vi "Writeini.vi"(10 "Number Sample for avarage AF":i32, 11 "data":waveform(dbl)[](array[waveform])) -> ()   [LabVIEW 2017]
uses:
  <vilib>/measure/matone.llb/Harmonic Distortion Analyzer N Chan.vi
  <vilib>/measure/matone.llb/Extract Single Tone Information N Chan.vi
  <vilib>/Utility/config.llb/Write Key (Double).vi
  <vilib>/Utility/config.llb/Write Key (Boolean).vi
  <vilib>/Utility/config.llb/NI_LVConfig.lvlib
  <vilib>/measure/NI_MAPro.lvlib
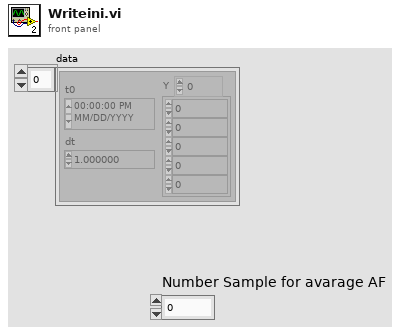
[diagram p1: front panel]
types:
  T1 = typedef "NI_LVConfig.lvlib/Config Data RefNum.ctl" = refnum<k1>
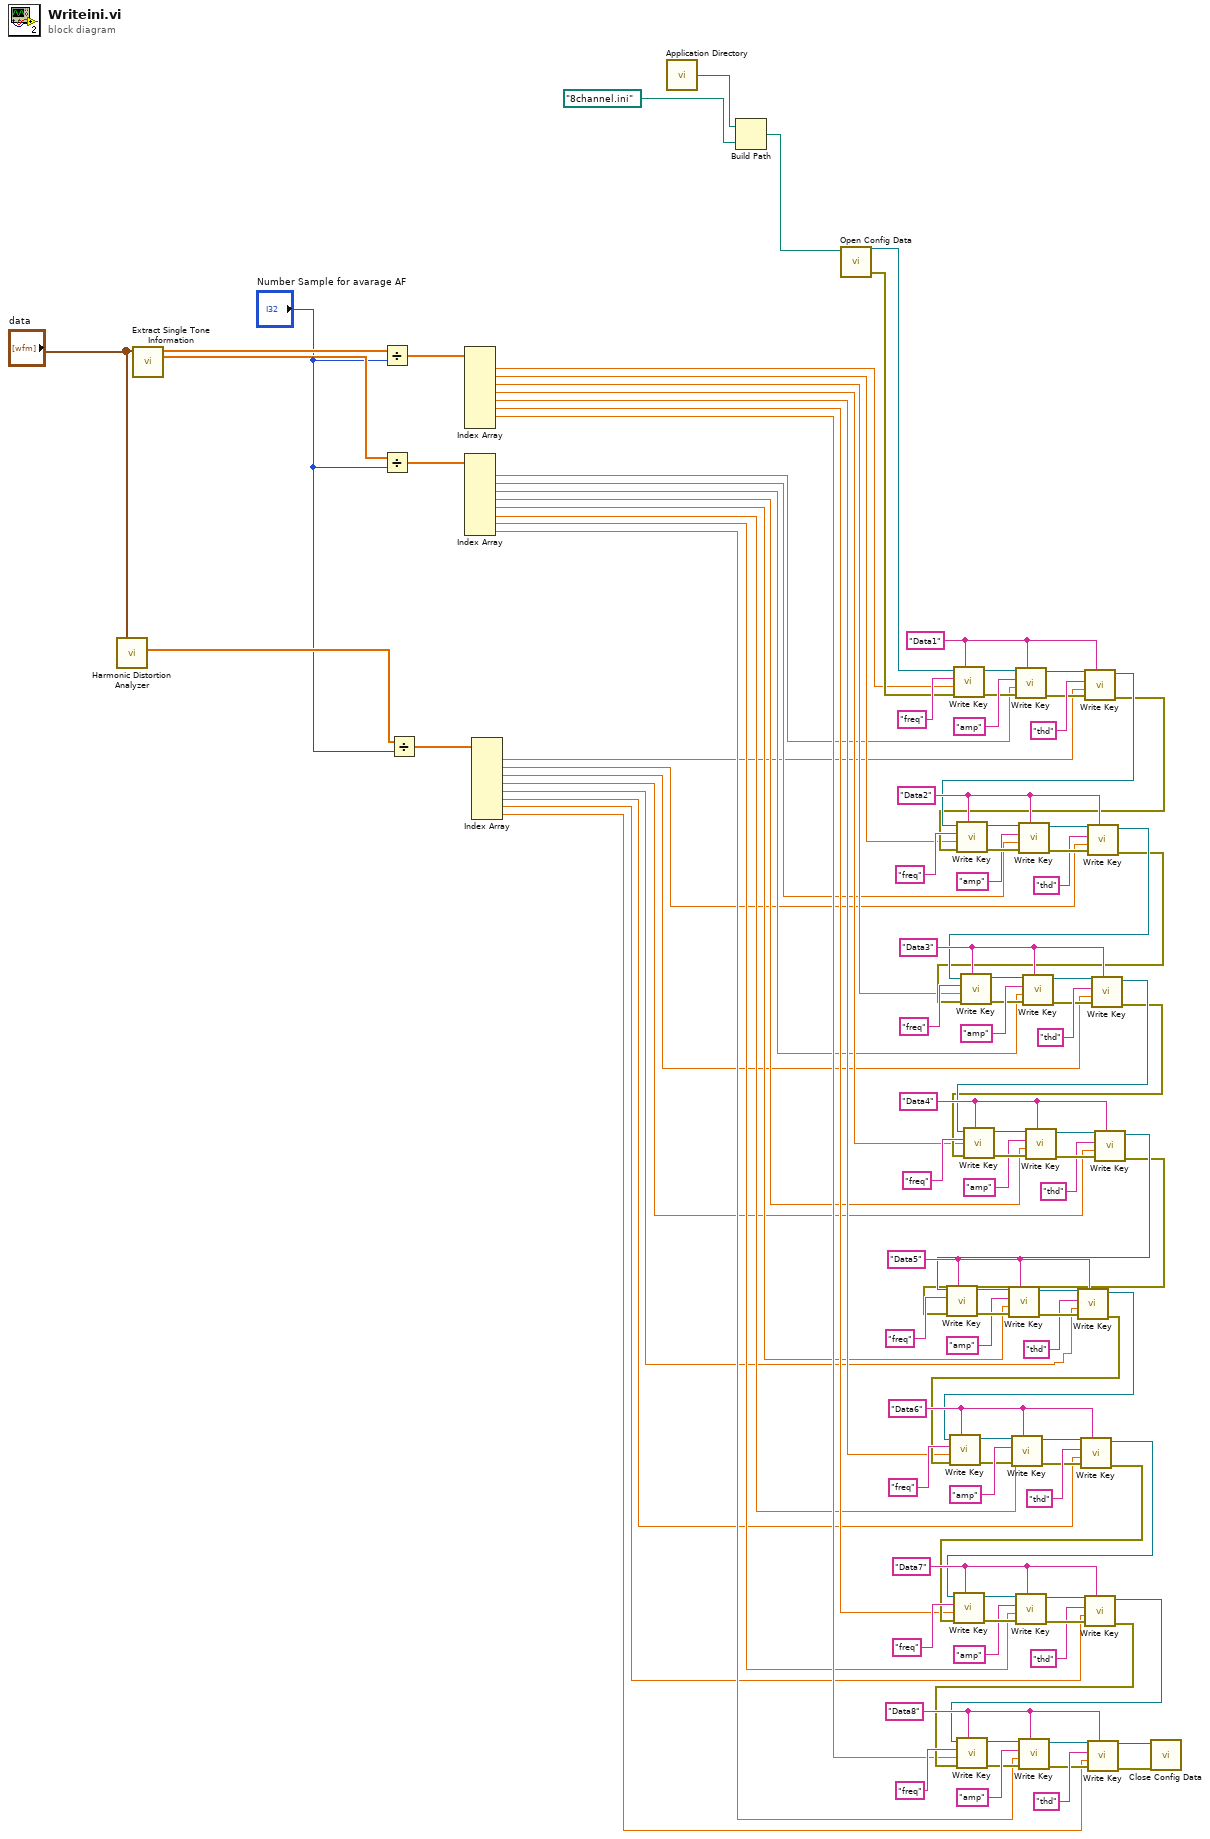
[diagram p0: block diagram]
diagram:
  w80 = "Data8" ("section")
  w65 = "Data7" ("section")
  w64 = "Data6" ("section")
  w49 = "Data5" ("section")
  w81 = "Data4" ("section")
  w96 = "Data3" ("section")
  w97 = "Data2" ("section")
  w113 = "Data1" ("section")
  n1 = call-poly <vilib>:"Harmonic Distortion Analyzer.vi"("signals in"="data") -> ("THD"=w10:dbl[])  [unwired: 5 in, 5 out]
  n2 = call-poly <vilib>:"Extract Single Tone Information.vi"("time signals in"="data") -> ("detected amplitudes"=w20:dbl[], "detected frequencies"=w21:dbl[])  [unwired: 5 in, 4 out]
  n3 = Divide(x=w21, y="Number Sample for avarage AF") -> (x/y=w23:dbl[])
  n4 = Divide(x=w20, y="Number Sample for avarage AF") -> (x/y=w22:dbl[])
  n5 = Divide(x=w10, y="Number Sample for avarage AF") -> (x/y=w11:dbl[])
  n6 = Index Array(array=w23) -> (element #1=w33:dbl, element #2=w32:dbl, element #3=w31:dbl, element #4=w29:dbl, element #5=w28:dbl, element #6=w27:dbl, element #7=w26:dbl)  [unwired: 8 in, 1 out]
  n7 = Index Array(array=w22) -> (element #1=w19:dbl, element #2=w18:dbl, element #3=w17:dbl, element #4=w16:dbl, element #5=w15:dbl, element #6=w14:dbl, element #7=w13:dbl, element #8=w12:dbl)  [unwired: 8 in]
  n8 = Index Array(array=w11) -> (element #1=w8:dbl, element #2=w7:dbl, element #3=w6:dbl, element #4=w5:dbl, element #5=w4:dbl, element #6=w3:dbl, element #7=w2:dbl, element #8=w1:dbl)  [unwired: 8 in]
  n9 = call <vilib>:"Application Directory.vi"() -> ("Application Directory"=w114:path)
  n10 = Build Path(base path=w114, name or relative path=path "8channel.ini" ("appended path")) -> (appended path=w105:path)
  n11 = call <vilib>:"Open Config Data.vi"("configuration file path"=w105) -> ("error out"=w47:errorcluster, "refnum"=w48:T1)  [unwired: 8 in, 1 out]
  n12 = call-poly <vilib>:"Write Key.vi"("section"=w113, "error in (no error)"=w47, "value"=w33, "key"="freq", "refnum"=w48) -> ("error out"=w107:errorcluster, "refnum out"=w106:T1)  [unwired: 4 in, 1 out]
  n13 = call-poly <vilib>:"Write Key.vi"("section"=w113, "error in (no error)"=w107, "value"=w19, "key"="amp", "refnum"=w106) -> ("error out"=w111:errorcluster, "refnum out"=w110:T1)  [unwired: 4 in, 1 out]
  n14 = call-poly <vilib>:"Write Key.vi"("section"=w113, "error in (no error)"=w111, "value"=w8, "key"="thd", "refnum"=w110) -> ("error out"=w45:errorcluster, "refnum out"=w46:T1)  [unwired: 4 in, 1 out]
  n15 = call-poly <vilib>:"Write Key.vi"("section"=w97, "error in (no error)"=w45, "value"=w32, "key"="freq", "refnum"=w46) -> ("error out"=w103:errorcluster, "refnum out"=w104:T1)  [unwired: 4 in, 1 out]
  n16 = call-poly <vilib>:"Write Key.vi"("section"=w97, "error in (no error)"=w103, "value"=w18, "key"="amp", "refnum"=w104) -> ("error out"=w99:errorcluster, "refnum out"=w100:T1)  [unwired: 4 in, 1 out]
  n17 = call-poly <vilib>:"Write Key.vi"("section"=w97, "error in (no error)"=w99, "value"=w7, "key"="thd", "refnum"=w100) -> ("error out"=w43:errorcluster, "refnum out"=w44:T1)  [unwired: 4 in, 1 out]
  n18 = call-poly <vilib>:"Write Key.vi"("section"=w96, "error in (no error)"=w43, "value"=w31, "key"="freq", "refnum"=w44) -> ("error out"=w90:errorcluster, "refnum out"=w89:T1)  [unwired: 4 in, 1 out]
  n19 = call-poly <vilib>:"Write Key.vi"("section"=w96, "error in (no error)"=w90, "value"=w17, "key"="amp", "refnum"=w89) -> ("error out"=w94:errorcluster, "refnum out"=w93:T1)  [unwired: 4 in, 1 out]
  n20 = call-poly <vilib>:"Write Key.vi"("section"=w96, "error in (no error)"=w94, "value"=w6, "key"="thd", "refnum"=w93) -> ("error out"=w30:errorcluster, "refnum out"=w42:T1)  [unwired: 4 in, 1 out]
  n21 = call-poly <vilib>:"Write Key.vi"("section"=w81, "error in (no error)"=w30, "value"=w29, "key"="freq", "refnum"=w42) -> ("error out"=w87:errorcluster, "refnum out"=w88:T1)  [unwired: 4 in, 1 out]
  n22 = call-poly <vilib>:"Write Key.vi"("section"=w81, "error in (no error)"=w87, "value"=w16, "key"="amp", "refnum"=w88) -> ("error out"=w83:errorcluster, "refnum out"=w84:T1)  [unwired: 4 in, 1 out]
  n23 = call-poly <vilib>:"Write Key.vi"("section"=w81, "error in (no error)"=w83, "value"=w5, "key"="thd", "refnum"=w84) -> ("error out"=w40:errorcluster, "refnum out"=w41:T1)  [unwired: 4 in, 1 out]
  n24 = call-poly <vilib>:"Write Key.vi"("section"=w49, "error in (no error)"=w40, "key"="freq", "refnum"=w41) -> ("error out"=w55:errorcluster, "refnum out"=w56:T1)  [unwired: 5 in, 1 out]
  n25 = call-poly <vilib>:"Write Key.vi"("section"=w49, "error in (no error)"=w55, "value"=w15, "key"="amp", "refnum"=w56) -> ("error out"=w51:errorcluster, "refnum out"=w52:T1)  [unwired: 4 in, 1 out]
  n26 = call-poly <vilib>:"Write Key.vi"("section"=w49, "error in (no error)"=w51, "value"=w4, "key"="thd", "refnum"=w52) -> ("error out"=w36:errorcluster, "refnum out"=w39:T1)  [unwired: 4 in, 1 out]
  n27 = call-poly <vilib>:"Write Key.vi"("section"=w64, "error in (no error)"=w36, "value"=w28, "key"="freq", "refnum"=w39) -> ("error out"=w58:errorcluster, "refnum out"=w57:T1)  [unwired: 4 in, 1 out]
  n28 = call-poly <vilib>:"Write Key.vi"("section"=w64, "error in (no error)"=w58, "value"=w14, "key"="amp", "refnum"=w57) -> ("error out"=w62:errorcluster, "refnum out"=w61:T1)  [unwired: 4 in, 1 out]
  n29 = call-poly <vilib>:"Write Key.vi"("section"=w64, "error in (no error)"=w62, "value"=w3, "key"="thd", "refnum"=w61) -> ("error out"=w35:errorcluster, "refnum out"=w38:T1)  [unwired: 4 in, 1 out]
  n30 = call-poly <vilib>:"Write Key.vi"("section"=w65, "error in (no error)"=w35, "value"=w27, "key"="freq", "refnum"=w38) -> ("error out"=w71:errorcluster, "refnum out"=w72:T1)  [unwired: 4 in, 1 out]
  n31 = call-poly <vilib>:"Write Key.vi"("section"=w65, "error in (no error)"=w71, "value"=w13, "key"="amp", "refnum"=w72) -> ("error out"=w67:errorcluster, "refnum out"=w68:T1)  [unwired: 4 in, 1 out]
  n32 = call-poly <vilib>:"Write Key.vi"("section"=w65, "error in (no error)"=w67, "value"=w2, "key"="thd", "refnum"=w68) -> ("error out"=w34:errorcluster, "refnum out"=w37:T1)  [unwired: 4 in, 1 out]
  n33 = call-poly <vilib>:"Write Key.vi"("section"=w80, "error in (no error)"=w34, "value"=w26, "key"="freq", "refnum"=w37) -> ("error out"=w74:errorcluster, "refnum out"=w73:T1)  [unwired: 4 in, 1 out]
  n34 = call-poly <vilib>:"Write Key.vi"("section"=w80, "error in (no error)"=w74, "value"=w12, "key"="amp", "refnum"=w73) -> ("error out"=w78:errorcluster, "refnum out"=w77:T1)  [unwired: 4 in, 1 out]
  n35 = call-poly <vilib>:"Write Key.vi"("section"=w80, "error in (no error)"=w78, "value"=w1, "key"="thd", "refnum"=w77) -> ("error out"=w24:errorcluster, "refnum out"=w25:T1)  [unwired: 4 in, 1 out]
  n36 = call <vilib>:"Close Config Data.vi"("error in (no error)"=w24, "refnum"=w25) -> ()  [unwired: 8 in, 2 out]
